vi "filtro Adaptativo LV ECG por lotes.vi"() -> ()   [LabVIEW 2014]
doc: "This example demonstrates how to extract fetal electrocardiogram (ECG) signals from maternal abdominal ECG signals. You obtain maternal abdominal ECG signals from obdominal leads. Maternal abdominal ECG signals contain both maternal ECG signals and fetal ECG signals. You can use an adaptive filter to extract fetal ECG signals from maternal abdominal ECG signals. To use an adaptive filter as the solution, you must obtain maternal thorax ECG signals from thorax leads as reference signals."
uses:
  Documents/sd_2015_2/Control 1.ctl
  <vilib>/addons/Adaptive Filters/Create/AFT Create FIR LMS (Real).vi
  <vilib>/addons/Adaptive Filters/Processing/AFT Filter Signal and Update Coefficients (Real, Array).vi
  <vilib>/addons/Adaptive Filters/NI_AdaptiveFilter.lvlib
  <vilib>/Analysis/NI_AALBase.lvlib
panel:
  in  "Rata de convegencia":T1=0.45 min=0.0 step=0.01 format="%#_9f"
  in  "longitud del filtro":i32=40 min=2
  out "señal de salida":dbl[](graph)
  out "señal de entrada":dbl[](graph)
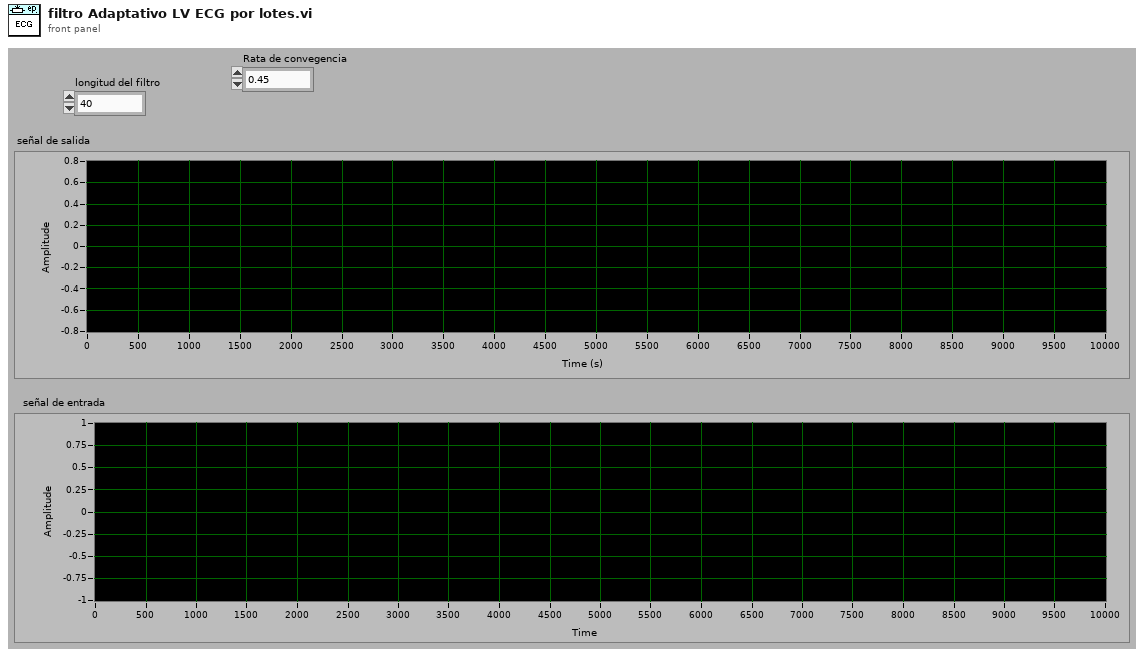
[diagram p1: front panel]
types:
  T1 = typedef "Control 1.ctl" = dbl
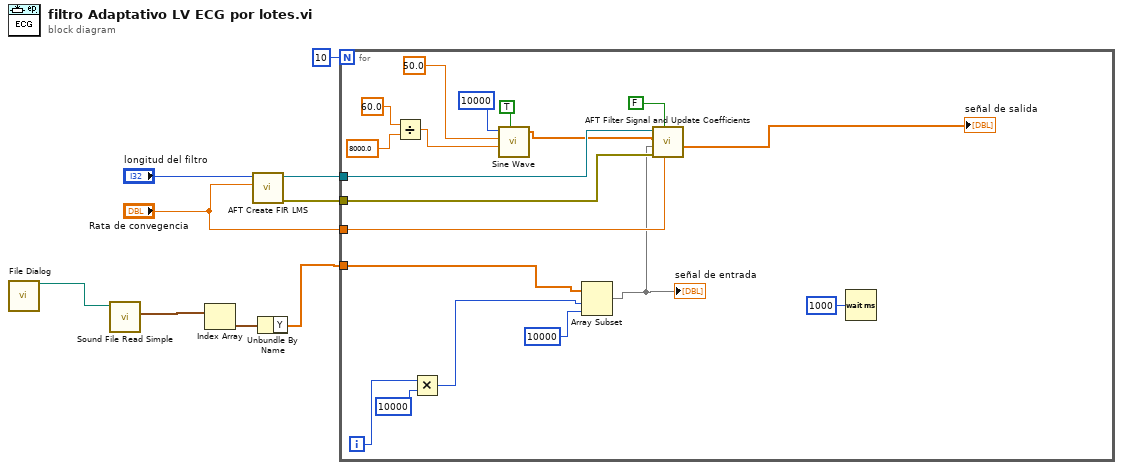
[diagram p0: block diagram]
diagram:
  n1 = call "File Dialog"() -> ("selected path"=w5:path)  [unwired: 12 in, 3 out]
  n2 = call <vilib>:"Sound File Read Simple.vi"("path"=w5) -> ("data"=w4:waveform(dbl)[])  [unwired: 7 in, 3 out]
  n3 = Index Array(array=w4) -> (element=w3:waveform(dbl))  [unwired: 1 in]
  n4 = call-poly <vilib>:"AFT Create FIR LMS.vi"("step size"="Rata de convegencia", "filter length"="longitud del filtro") -> ("error out"=w6:errorcluster, "adaptive filter out"=w7:refnum<k20>)  [unwired: 2 in, 6 out]
  n5 = Unbundle By Name(w3) -> ("Y"=w2:dbl[])
  n6 = for {
    N: 10 -> [_]
    tunnel: w2 -> [w27]
    tunnel: w7 -> [w16]
    tunnel: w6 -> [w15]
    tunnel: "Rata de convegencia" -> [w14]
    i -> [w26]
    n7 = Divide(x=60.0, y=8000.0) -> (x/y=w19:dbl)
    n8 = Multiply(x=w26, y=10000) -> (x*y=w24:i32)
    n9 = call <vilib>:"Sine Wave.vi"("samples"=10000, "amplitude"=50.0, "frequency"=w19, "reset phase"=TRUE) -> ("sine wave"=w11:dbl[])  [unwired: 1 in, 2 out]
    n10 = Array Subset(array=w27, index=w24, length=10000) -> (w10:dbl[])
    "señal de entrada" <- w10
    n11 = call-poly <vilib>:"AFT Filter Signal and Update Coefficients.vi"("step size"=w14, "reset? (F)"=FALSE, "error in (no error)"=w15, "d(n)"=w10, "x(n)"=w11, "adaptive filter in"=w16) -> ("e(n)"=→"señal de salida":dbl[])  [unwired: 5 out]
    n12 = Wait (ms)(milliseconds to wait=u32 1000) -> ()  [unwired: 1 out]
  }
